vi "MC LV Link3 with DIO Hack Engine.vi"(0 "Unique Notifier Name":string="Not a Name", 11 "AO Chn and Limits":string[](array[string])) -> ()   [LabVIEW 2016]
uses:
  External Power Control Type Defs/External Power Notifier Type.ctl
  External Power Control Type Defs/External Power Actions.ctl
  <userlib>/LV-Link3/PolySubVIs/DtCreateAoutChan.vi
  <userlib>/LV-Link3/PolySubVIs/DtOLWriteSingle.vi
panel:
  in  "Power (%)":dbl
  in  "Quit":bool
  in  "Line On Off":bool
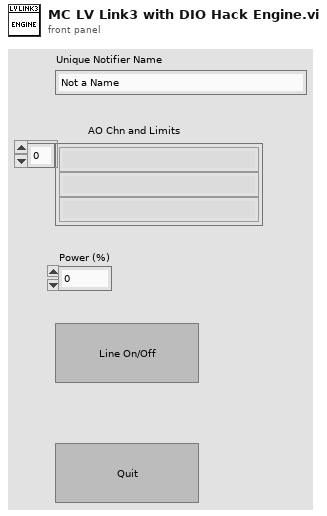
[diagram p1: front panel]
types:
  T1 = typedef "External Power Notifier Type.ctl" = cluster{"Actions":T2, "Wavelength":string, "Line On/Off":bool, "Power (%)":dbl, "Control Parameters":variant, "Cmd Done?":bool}
  T2 = typedef "External Power Actions.ctl" = enum16{"Line On/Off", "Set Power", "Set Ctrl Parameters", "Quit"}
  T3 = enum32{"Invalid", "Standard", "Closed", "Hidden", "Minimized", "Maximized"}
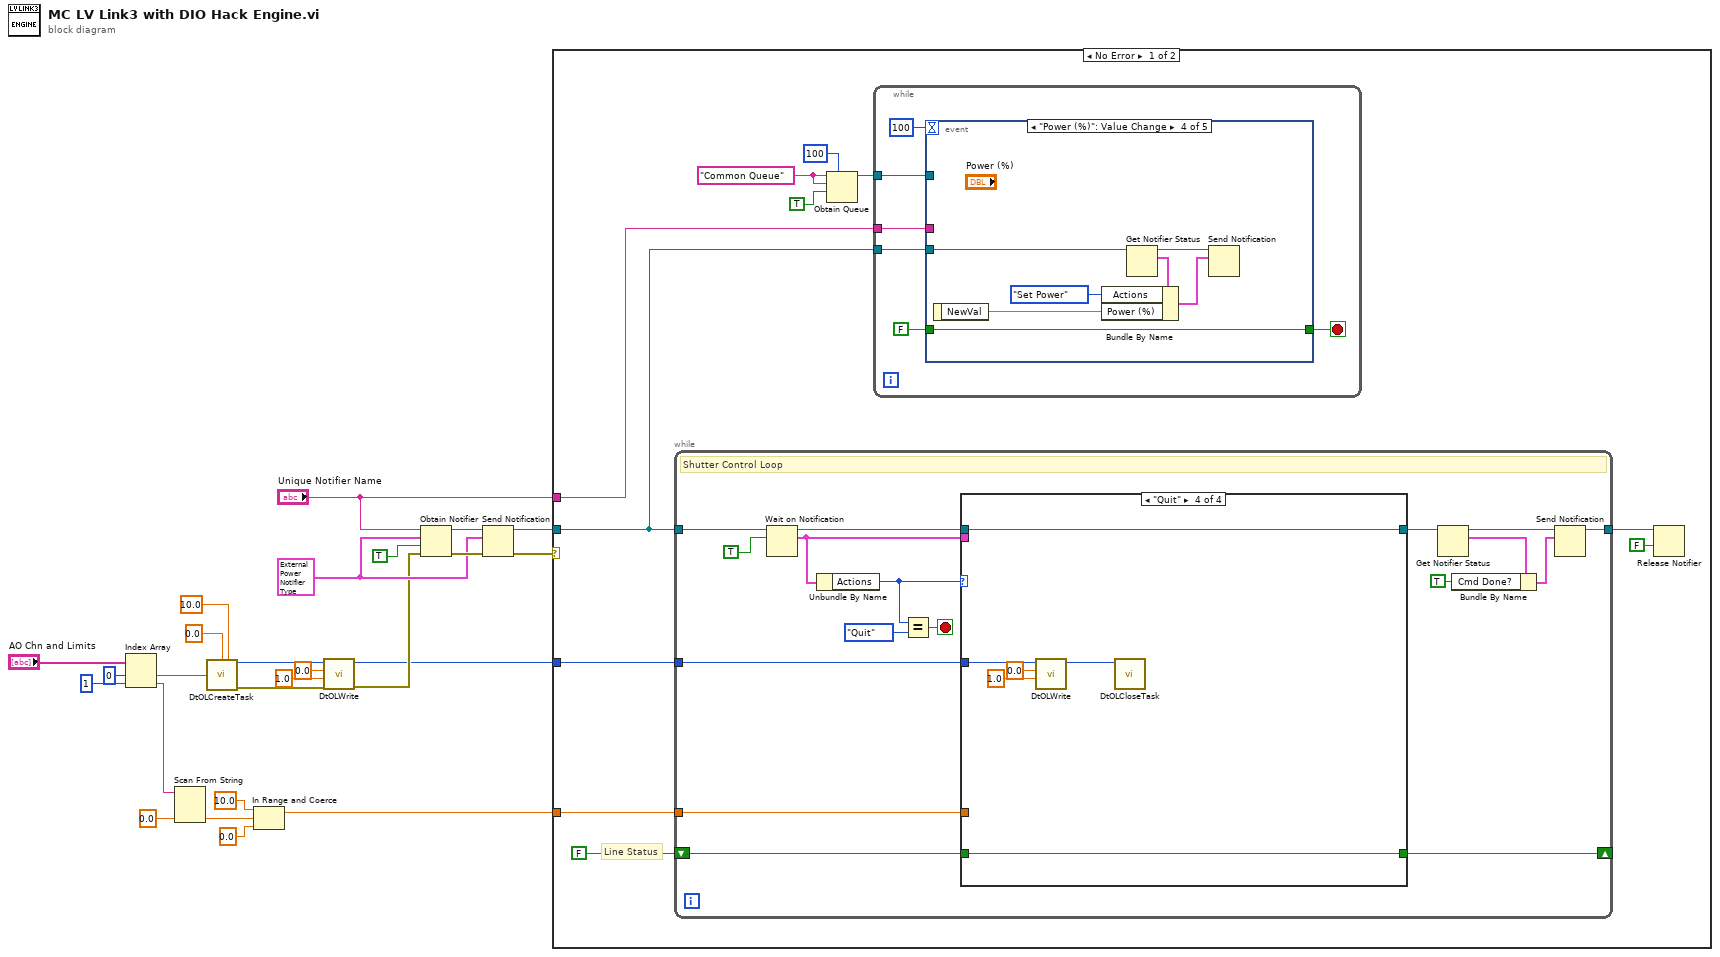
[diagram p0: block diagram]
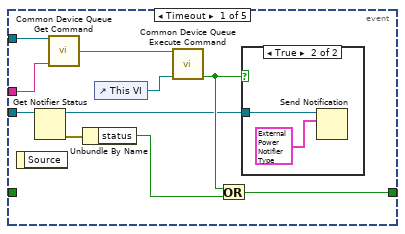
[diagram p2: hidden frame]
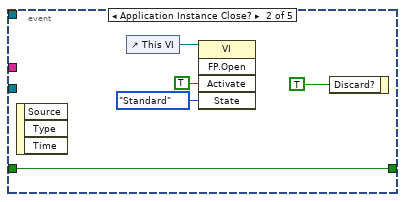
[diagram p4: hidden frame]
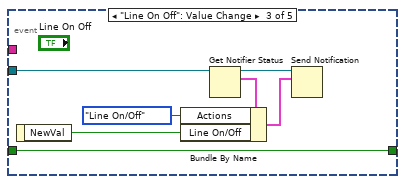
[diagram p5: hidden frame]
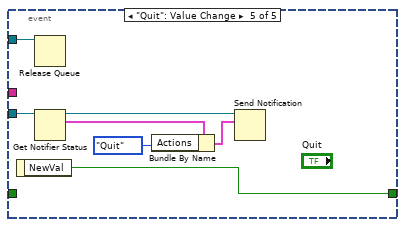
[diagram p6: hidden frame]
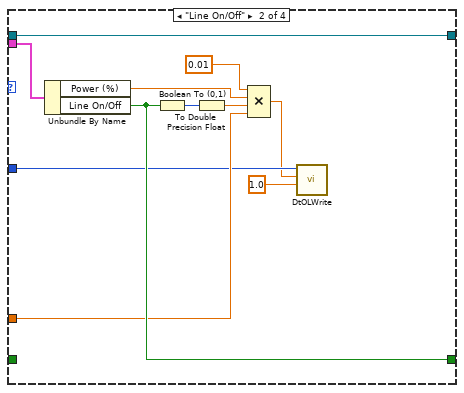
[diagram p8: hidden frame]
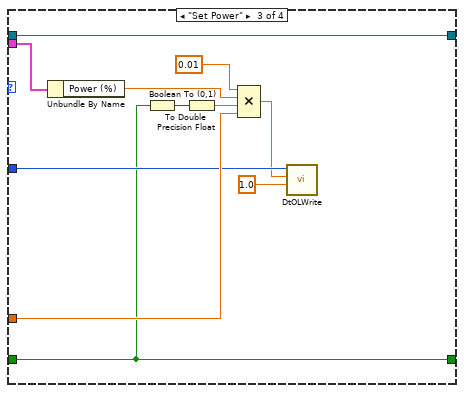
[diagram p9: hidden frame]
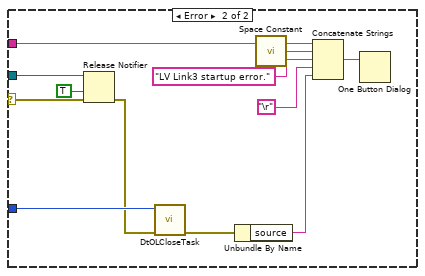
[diagram p10: hidden frame]
diagram:
  w21 = T1 {"Actions"=enum."Set Power", "Wavelength"="", "Line On/Off"=FALSE, "Power (%)"=0.0, "Control Parameters"=variant, "Cmd Done?"=FALSE} ("External Ctrl")
  n1 = Index Array(array="AO Chn and Limits", index #1=0 ("index"), index #2=1 ("index")) -> (element #1=w17:string, element #2=w2:string)
  n2 = Scan From String(input string=w2, default 1=0.0 ("default value 1")) -> (output 1=w6:dbl)  [unwired: 3 in, 3 out]
  n3 = call-poly <userlib>:"DtOLCreateTask.vi"("Range Min"=0.0, "Range Max"=10.0, "Channel"=w17) -> ("Task out"=w15:i32, "error out"=w14:errorcluster)  [unwired: 10 in, 1 out]
  n4 = In Range and Coerce(upper limit=10.0, x=w6, lower limit=0.0) -> (coerced(x)=w1:dbl)  [unwired: 1 out]
  n5 = call-poly <userlib>:"DtOLWrite.vi"("error in (no error)"=w14, "Timeout"=1.0, "Data In"=0.0, "Task in"=w15) -> ("error out"=w12:errorcluster, "Task out"=w11:i32)  [unwired: 6 in]
  n6 = Obtain Notifier(name (unnamed)="Unique Notifier Name", notification data type=w21, create if not found? (T)=TRUE, error in (no error)=w12) -> (notifier out=w24:refnum<notifier>, error out=w23:errorcluster)  [unwired: 1 out]
  n7 = Send Notification(notification=w21, notifier=w24, error in (no error)=w23) -> (notifier out=w22:refnum<notifier>, error out=w20:errorcluster)
  n8 = case shown="No Error" w20 {
    selector: w20 -> [_ w137]
    tunnel: w11 -> [w36 w130]
    tunnel: w22 -> [w34 w138]
    tunnel: "Unique Notifier Name" -> [w33 w136]
    tunnel: w1 -> [w27 _]
    frame No Error {
      w32 = "Common Queue" ("Unique Notifier Name")
      # "Line Status"
      n9 = while {
        tunnel: w34 -> [w89]
        tunnel: w36 -> [w95]
        tunnel: [w90] -> w26
        shift-right: [w82] -> _
        shift-left: FALSE -> [w83]
        tunnel: w27 -> [w81]
        stop <- w96 stop-if-true
        # "Shutter Control Loop"
        n10 = Wait on Notification(notifier=w89, ignore previous (F)=TRUE) -> (notifier out=w88:refnum<notifier>, notification=w87:T1)  [unwired: 2 in, 2 out]
        n11 = Unbundle By Name(w87) -> ("Actions"=w86:T2)
        n12 = Equal?(x=w86, y=External_Power_Actions."Quit") -> (x = y?=w96:bool)
        n13 = case shown="\"Quit\"" w86 {
          tunnel: w88 -> [w99 w110 w121 w127]
          tunnel: w95 -> [_ w101 w113 w123]
          tunnel: [w99 w110 w121 w127] -> w93
          tunnel: w87 -> [_ w109 w120 _]
          tunnel: w83 -> [w98 _ w111 w126]
          tunnel: [w98 w107 w111 w126] -> w82
          tunnel: w81 -> [_ w103 w115 _]
          frame Default {
          }
          frame "Line On/Off" {
            n14 = Unbundle By Name(w109) -> ("Power (%)"=w105:dbl, "Line On/Off"=w107:bool)
            n15 = Boolean To (0,1)(Boolean=w107) -> (0, 1=w108:i16)
            n16 = To Double Precision Float(number=w108) -> (double precision float=w106:dbl)
            n17 = Compound Arithmetic op=MULTIPLY(0.01 ("value"), w105, w106, w103) -> (w100:dbl)
            n18 = call-poly <userlib>:"DtOLWrite.vi"("Timeout"=1.0, "Data In"=w100, "Task in"=w101) -> ()  [unwired: 7 in, 2 out]
          }
          frame "Set Power" {
            n19 = Unbundle By Name(w120) -> ("Power (%)"=w117:dbl)
            n20 = Boolean To (0,1)(Boolean=w111) -> (0, 1=w119:i16)
            n21 = To Double Precision Float(number=w119) -> (double precision float=w118:dbl)
            n22 = Compound Arithmetic op=MULTIPLY(0.01 ("value"), w117, w118, w115) -> (w112:dbl)
            n23 = call-poly <userlib>:"DtOLWrite.vi"("Timeout"=1.0, "Data In"=w112, "Task in"=w113) -> ()  [unwired: 7 in, 2 out]
          }
          frame "Quit" {
            n24 = call-poly <userlib>:"DtOLWrite.vi"("Timeout"=1.0, "Data In"=0.0, "Task in"=w123) -> ("Task out"=w122:i32)  [unwired: 7 in, 1 out]
            n25 = call <userlib>:"DtOLCloseTask.vi"("Task in"=w122) -> ()  [unwired: 10 in, 1 out]
          }
        }
        n26 = Get Notifier Status(notifier=w93) -> (notifier out=w91:refnum<notifier>, current notification=w94:T1)  [unwired: 1 in, 3 out]
        n27 = Bundle By Name(cluster=w94, "Cmd Done?"=TRUE ("Received?")) -> (w84:T1)
        n28 = Send Notification(notification=w84, notifier=w91) -> (notifier out=w90:refnum<notifier>)  [unwired: 1 in, 1 out]
      }
      n29 = Obtain Queue(max queue size (-1, unlimited)=100, name (unnamed)=w32, element data type=w32, create if not found? (T)=TRUE) -> (queue out=w29:refnum<queue>)  [unwired: 1 in, 2 out]
      n30 = while {
        tunnel: w29 -> [w42]
        tunnel: w34 -> [w39]
        tunnel: w33 -> [w37]
        stop <- w38 stop-if-true
        n31 = event shown="[3] \"Power (%)\": Value Change" {
          selector: _ -> [_ _ _ _ _]
          dyn-events: _ -> [_ _ _ _ _]
          timeout: 100 -> [_ _ _ _ _]
          tunnel: w42 -> [w50 _ _ _ w75]
          tunnel: FALSE -> [_ w59 w62 w69 _]
          tunnel: w39 -> [w52 _ w66 w73 w76]
          tunnel: [w45 w59 w62 w69 w80] -> w38
          tunnel: w37 -> [w49 _ _ _ _]
          event Timeout {
            n32 = event-data() -> ()  [unwired: 1 in, 1 out]
            n33 = Get Notifier Status(notifier=w52) -> (notifier out=w43:refnum<notifier>, error out=w51:errorcluster)  [unwired: 1 in, 3 out]
            n34 = call "Common Device Queue Get Command.vi"("Common Queue"=w50, "Notifier Name"=w49) -> ("Command"=w48:string)  [unwired: 12 in, 1 out]
            n35 = Unbundle By Name(w51) -> ("status"=w46:bool)
            n36 = control-ref of="This VI"() -> (w47:refnum<vi>)
            n37 = call "Common Device Queue Execute Command.vi"("Common Command"=w48, "VI Refnum"=w47) -> ("Quit?"=w44:bool)  [unwired: 12 in, 1 out]
            n38 = Or(x=w44, y=w46) -> (x .or. y?=w45:bool)
            n39 = case shown="True" w44 {
              tunnel: w43 -> [_ w54]
              frame False {
              }
              frame True {
                n40 = Send Notification(notification=T1 {"Actions"=enum."Quit", "Wavelength"="", "Line On/Off"=FALSE, "Power (%)"=0.0, "Control Parameters"=variant, "Cmd Done?"=FALSE} ("External Ctrl"), notifier=w54) -> ()  [unwired: 1 in, 2 out]
              }
            }
          }
          event Application Instance Close? {
            n41 = event-data() -> ()  [unwired: 1 in, 3 out]
            n42 = control-ref of="This VI"() -> (w56:refnum<vi>)
            n43 = invoke class="VI" method="FP.Open"(reference=w56, "Activate"=TRUE ("Activate?"), "State"=T3."Standard") -> ()  [unwired: 2 in, 5 out]
            n44 = event-data("Discard?"=TRUE) -> ()  [unwired: 1 in, 1 out]
          }
          event "Line On Off": Value Change {
            n45 = event-data() -> ("NewVal"=w61:bool)  [unwired: 1 in]
            n46 = Get Notifier Status(notifier=w66) -> (notifier out=w65:refnum<notifier>, current notification=w64:T1)  [unwired: 1 in, 3 out]
            n47 = Bundle By Name(cluster=w64, "Actions"=External_Power_Actions."Line On/Off", "Line On/Off"=w61) -> (w63:T1)
            n48 = Send Notification(notification=w63, notifier=w65) -> ()  [unwired: 1 in, 2 out]
          }
          event "Power (%)": Value Change {
            n49 = event-data() -> ("NewVal"=w68:dbl)  [unwired: 1 in]
            n50 = Get Notifier Status(notifier=w73) -> (notifier out=w72:refnum<notifier>, current notification=w71:T1)  [unwired: 1 in, 3 out]
            n51 = Bundle By Name(cluster=w71, "Actions"=External_Power_Actions."Set Power", "Power (%)"=w68) -> (w70:T1)
            n52 = Send Notification(notification=w70, notifier=w72) -> ()  [unwired: 1 in, 2 out]
          }
          event "Quit": Value Change {
            n53 = event-data() -> ("NewVal"=w80:bool)  [unwired: 1 in]
            n54 = Release Queue(queue=w75) -> ()  [unwired: 2 in, 3 out]
            n55 = Get Notifier Status(notifier=w76) -> (notifier out=w79:refnum<notifier>, current notification=w78:T1)  [unwired: 1 in, 3 out]
            n56 = Bundle By Name(cluster=w78, "Actions"=External_Power_Actions."Quit") -> (w77:T1)
            n57 = Send Notification(notification=w77, notifier=w79) -> ()  [unwired: 1 in, 2 out]
          }
        }
      }
      n58 = Release Notifier(notifier=w26, force destroy? (F)=FALSE) -> ()  [unwired: 1 in, 3 out]
    }
    frame Error {
      n59 = Release Notifier(notifier=w138, force destroy? (F)=TRUE, error in (no error)=w137) -> (error out=w128:errorcluster)  [unwired: 2 out]
      n60 = call <userlib>:"DtOLCloseTask.vi"("Error in"=w128, "Task in"=w130) -> ("Error Out"=w129:errorcluster)  [unwired: 9 in]
      n61 = Unbundle By Name(w129) -> ("source"=w131:string)
      n62 = call <vilib>:"Space Constant.vi"() -> ("String"=w134:string)
      n63 = Concatenate Strings(w136, w134, "LV Link3 startup error." ("string"), "\r", w131) -> (w135:string)
      n64 = One Button Dialog(message=w135) -> ()  [unwired: 1 in, 1 out]
    }
  }
